vi "Read Spectrum Analyzer.lvclass.vi"(11 "Switching Time in":refnum<class "Switching Time.lvclass">) -> (2 "Spectrum Analyzer.lvclass":refnum<class "Spectrum Analyzer.lvclass">, 3 "Switching Time out":refnum<class "Switching Time.lvclass">)   [LabVIEW 2020, in "Switching Time.lvclass"]
uses:
  Switching Time.lvclass
  Instruments/Spectrum Analyzer/Spectrum Analyzer.lvclass
  Switching Time.lvclass/Switching Time.ctl
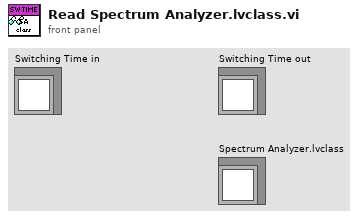
[diagram p1: front panel]
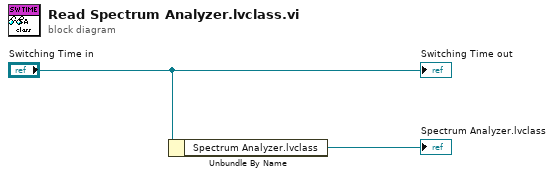
[diagram p0: block diagram]
diagram:
  n1 = Unbundle By Name("Switching Time in") -> ("Spectrum Analyzer.lvclass"=→"Spectrum Analyzer.lvclass":refnum<class "Spectrum Analyzer.lvclass">)
  "Switching Time out" <- "Switching Time in"
